vi "Do.vi"(8 "error in (no error)":errorcluster, 10 "Actor in":refnum<class "Actor.lvclass">, 11 "Reply Message":refnum<class "Reply Msg.lvclass">) -> (0 "error out":errorcluster, 2 "Actor out":refnum<class "Actor.lvclass">)   [LabVIEW 2013, in "Reply Msg.lvclass"]
uses:
  <vilib>/ActorFramework/Reply Msg/Reply Msg.lvclass
  <vilib>/ActorFramework/Actor/Actor.lvclass
  <vilib>/ActorFramework/Reply Msg/Reply Msg.lvclass/Reply Msg.ctl
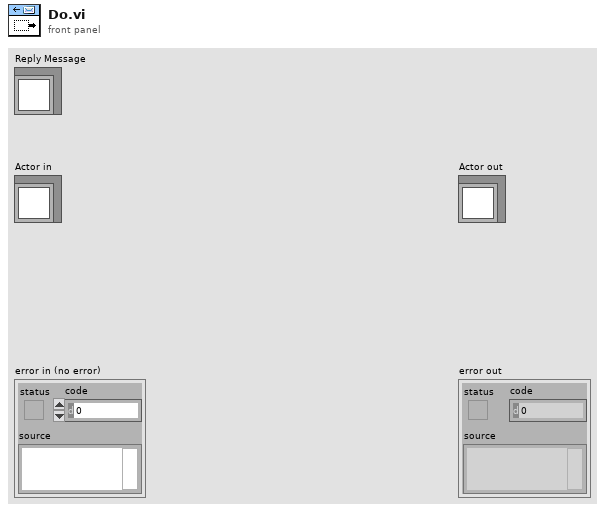
[diagram p1: front panel]
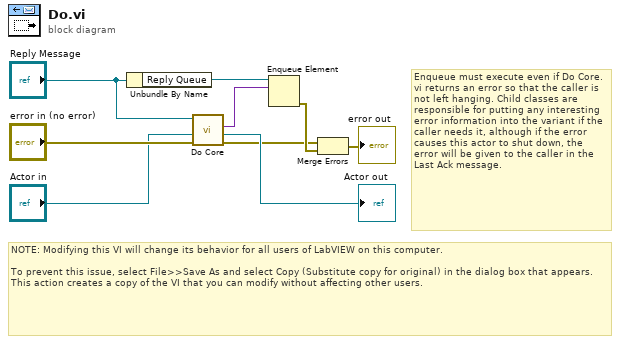
[diagram p0: block diagram]
diagram:
  # "Enqueue must execute even if Do Core.vi returns an error so that the caller is not left hanging. Child classes are responsible for putting any interesting error information into the variant if the caller needs it, although if the error causes this actor to shut down, the error will be given to the caller in the Last Ack message."
  # "NOTE: Modifying this VI will change its behavior for all users of LabVIEW on this computer.\n\nTo prevent this issue, select File>>Save As and select Copy (Substitute copy for original) in the dialog box that appears. This action creates a copy of the VI that you can modify without affecting other users."
  n1 = Unbundle By Name("Reply Message") -> ("Reply Queue"=w5:refnum<queue>)
  n2 = call-dynamic "Do Core.vi"("error in (no error)"="error in (no error)", "Actor in"="Actor in", "Reply Message"="Reply Message") -> ("error out"=w1:errorcluster, "Actor out"=→"Actor out":refnum<class "Actor.lvclass">, "Reply"=w4:variant)  [unwired: 6 in]
  n3 = Enqueue Element(queue=w5, element=w4) -> (error out=w2:errorcluster)  [unwired: 2 in, 2 out]
  n4 = Merge Errors(w1, w2) -> (→"error out":errorcluster)
